vi "Part 2.vi"(11 "Input":string) -> (3 "Output":i64)   [LabVIEW 2021]
uses:
  <userlib>/_OpenG.lib/string/string.llb/Convert EOLs (String)__ogtk.vi
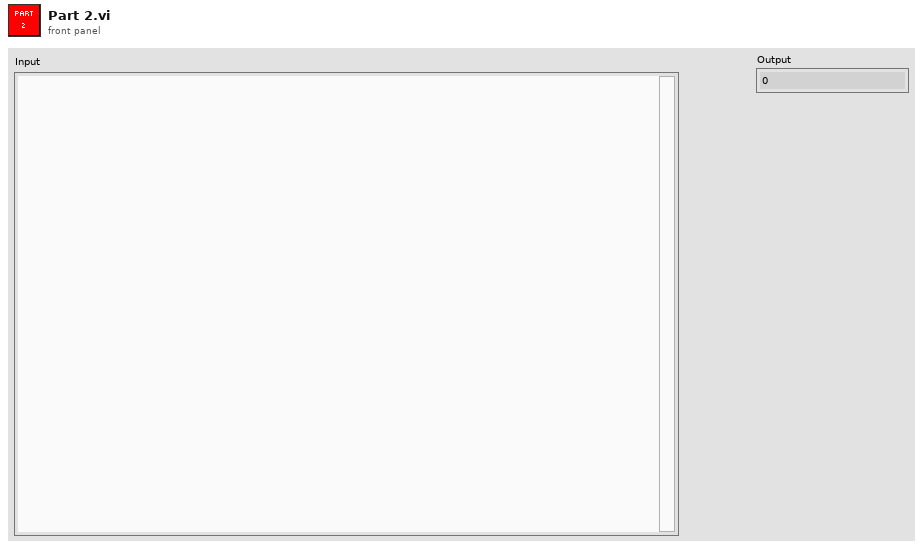
[diagram p1: front panel]
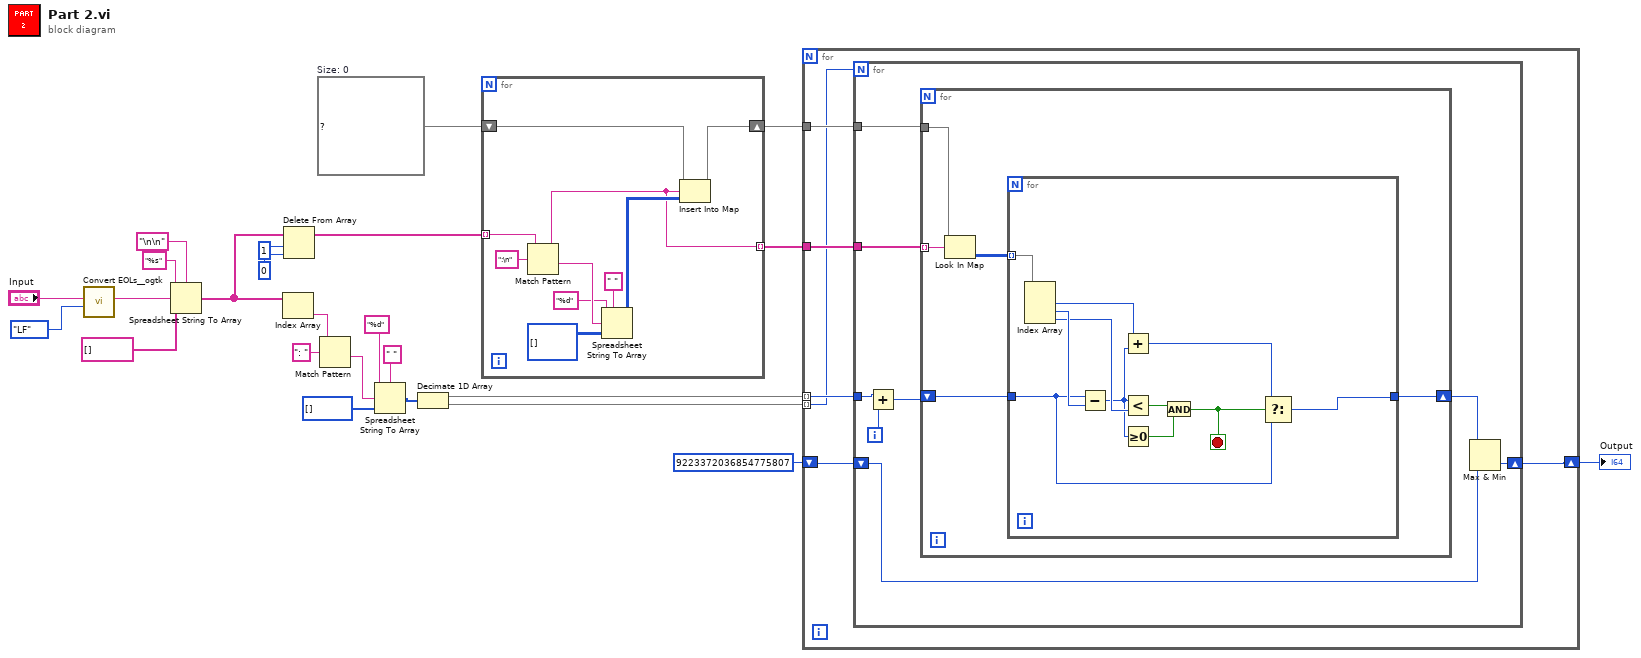
[diagram p0: block diagram]
diagram:
  w9 = map{string, i64[][]} {}  # Size: 0
  n1 = call-poly <userlib>:"Convert EOLs__ogtk.vi"("Convert to:"=enum16{"CR", "LF", "CRLF"}."LF", "String in"="Input") -> ("String out"=w20:string)  [unwired: 9 in]
  n2 = Spreadsheet String To Array(delimiter (Tab)="\n\n", format string="%s", spreadsheet string=w20, array type (2D Dbl)=string[] []) -> (array=w15:string[])
  n3 = Index Array(array=w15) -> (element=w14:string)  [unwired: 1 in]
  n4 = Delete From Array(array=w15, length=1, index=0) -> (array with subset deleted=w17:string[])  [unwired: 1 out]
  n5 = Match Pattern(string=w14, regular expression=": " ("search string/char (-)")) -> (after substring=w11:string)  [unwired: 1 in, 3 out]
  n6 = Spreadsheet String To Array(delimiter (Tab)=" ", format string="%d", spreadsheet string=w11, array type (2D Dbl)=i64[] []) -> (array=w5:i64[])
  n7 = Decimate 1D Array(w5) -> (w4:i64[], w3:i64[])
  n8 = for {
    tunnel: w17 -> [w33] mode=indexing
    shift-right: [w26] -> w7
    shift-left: w9 -> [w28]
    tunnel: [w25] -> w8 mode=indexing
    n9 = Match Pattern(string=w33, regular expression=":\n" ("search string/char (-)")) -> (before substring=w25:string, after substring=w31:string)  [unwired: 1 in, 2 out]
    n10 = Spreadsheet String To Array(delimiter (Tab)=" ", format string="%d", spreadsheet string=w31, array type (2D Dbl)=i64[][] []) -> (array=w27:i64[][])
    n11 = Insert Into Map(map in=w28, key=w25, value=w27) -> (map out=w26:map{string, i64[][]})  [unwired: 2 out]
  }
  n12 = for {
    tunnel: w4 -> [w38] mode=indexing
    tunnel: w8 -> [w40]
    tunnel: w7 -> [w39]
    tunnel: w3 -> [w35] mode=indexing
    shift-right: [w37] -> w2
    shift-left: i64 9223372036854775807 -> [w36]
    n13 = for {
      N: w35 -> [_]
      tunnel: w40 -> [w48]
      tunnel: w39 -> [w47]
      tunnel: w38 -> [w46]
      shift-right: [w42] -> w37
      shift-left: w36 -> [w41]
      i -> [w44]
      n14 = Add(x=w46, y=w44) -> (x+y=w45:i64)
      n15 = for {
        tunnel: w48 -> [w53] mode=indexing
        tunnel: w47 -> [w52]
        shift-right: [w49] -> w43
        shift-left: w45 -> [w50]
        n16 = Look In Map(map=w52, key=w53) -> (value=w51:i64[][])  [unwired: 1 in, 1 out]
        n17 = for {
          tunnel: w51 -> [w64] mode=indexing
          tunnel: w50 -> [w56]
          tunnel: [w54] -> w49
          stop <- w57 stop-if-true
          n18 = Index Array(array=w64) -> (element #1=w58:i64, element #2=w63:i64, element #3=w62:i64)  [unwired: 3 in]
          n19 = Subtract(x=w56, y=w63) -> (x-y=w59:i64)
          n20 = Add(x=w58, y=w59) -> (x+y=w55:i64)
          n21 = Less?(x=w59, y=w62) -> (x < y?=w61:bool)
          n22 = Greater Or Equal To 0?(x=w59) -> (x >= 0?=w60:bool)
          n23 = And(x=w61, y=w60) -> (x .and. y?=w57:bool)
          n24 = Select(t=w55, s=w57, f=w56) -> (s? t:f=w54:i64)
        }
      }
      n25 = Max & Min(x=w43, y=w41) -> (min(x,y)=w42:i64)  [unwired: 1 out]
    }
  }
  "Output" <- w2
